vi "Timestamp 1st.vi"(10 "subsystem":string, 11 "system":string) -> (2 "system timestamp":string)   [LabVIEW 2018]
panel:
  # "ISO 8601:\nSeptember 27, 2022 at 6 p.m. is represented as 2022-09-27 18:00:00.000."
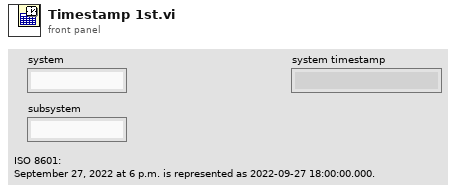
[diagram p1: front panel]
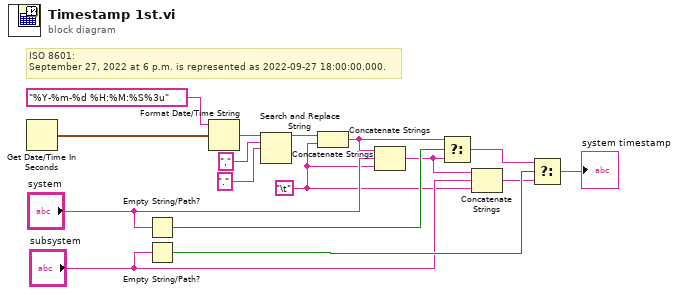
[diagram p0: block diagram]
diagram:
  w2 = "\t"
  # "ISO 8601:\nSeptember 27, 2022 at 6 p.m. is represented as 2022-09-27 18:00:00.000."
  n1 = Get Date/Time In Seconds() -> (seconds since 1Jan1904=w12:timestamp)
  n2 = Empty String/Path?(string/path="system") -> (empty?=w10:bool)
  n3 = Empty String/Path?(string/path="subsystem") -> (empty?=w8:bool)
  n4 = Format Date/Time String(time format string (%c)="%Y-%m-%d %H:%M:%S%3u", seconds (now)=w12) -> (date/time string=w15:string)  [unwired: 1 in]
  n5 = Search and Replace String(input string=w15, search string=",", replace string=".") -> (result string=w11:string)  [unwired: 5 in, 3 out]
  n6 = Concatenate Strings(w11, w2) -> (w9:string)
  n7 = Concatenate Strings(w9, "system", w2) -> (w4:string)
  n8 = Select(t=w9, s=w10, f=w4) -> (s? t:f=w7:string)
  n9 = Concatenate Strings(w4, "subsystem", w2) -> (w1:string)
  n10 = Select(t=w7, s=w8, f=w1) -> (s? t:f=→"system timestamp":string)
